vi "_060.vi"() -> ()   [LabVIEW 2024]
uses:
  <vilib>/Utility/file.llb/Read Delimited Spreadsheet (string).vi
panel:
  out "number":i32[][](array[numeric])
  in  "index 2":i32
  in  "index":i32
  out "all rows 2":string[][](array[string])
  in  "number of rows (all:-1)":i32=-1
  in  "disabled index (col) 2":i32
  out "subarray 2":string[](array[string])
  out "subarray":string[](array[string])
  in  "disabled index (col)":i32
  out "error out":errorcluster
  out "all rows":string[][](array[string])
  in  "file path (dialog if empty)":path
  # "Read Deliminated SpreadSheet :"
  # "( File IO )"
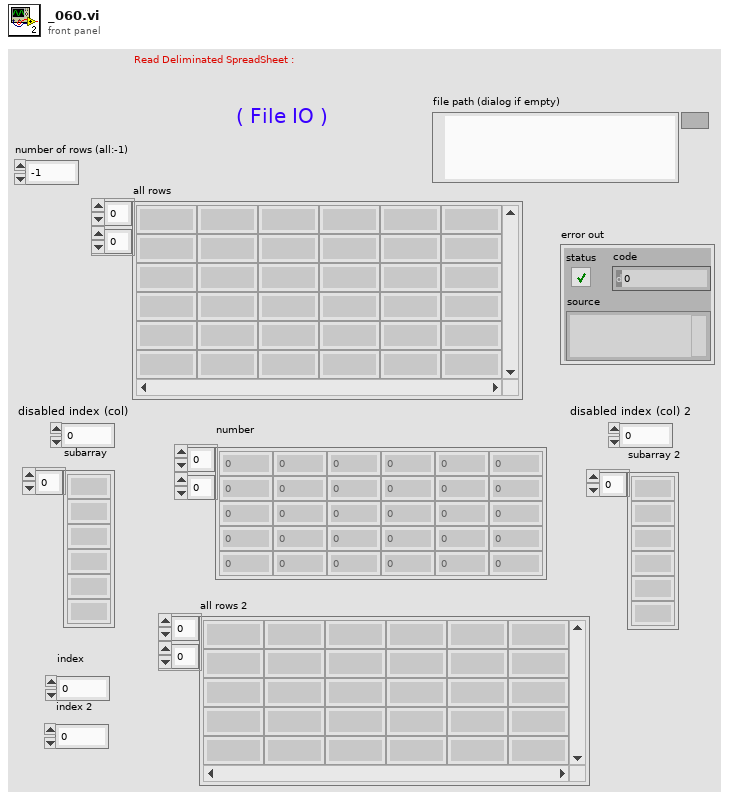
[diagram p1: front panel]
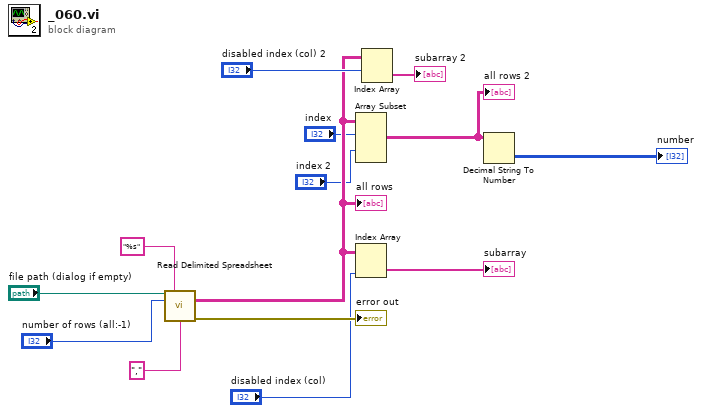
[diagram p0: block diagram]
diagram:
  n1 = call-poly <vilib>:"Read Delimited Spreadsheet.vi"("file path (dialog if empty)"="file path (dialog if empty)", "format (%s)"="%s", "number of rows (all:-1)"="number of rows (all:-1)", "delimiter (\\t)"="," ("delimiter (\\t)")) -> ("all rows"=w5:string[][], "error out"=→"error out":errorcluster)  [unwired: 6 in, 4 out]
  "all rows" <- w5
  n2 = Array Subset "Array Subset"(array=w5, index (row)="index", index (col)="index 2") -> (w2:string[][])  [unwired: 2 in]
  "all rows 2" <- w2
  n3 = Index Array "Index Array"(array=w5, index (col)="disabled index (col)") -> (element=→"subarray":string[])  [unwired: 1 in]
  n4 = Index Array(array=w5, index (row)="disabled index (col) 2") -> (element=→"subarray 2":string[])  [unwired: 1 in]
  n5 = Decimal String To Number(string=w2) -> (number=→"number":i32[][])  [unwired: 2 in, 1 out]
